vi "Fire WD Event.vi"(8 "error in (no error)":errorcluster, 10 "Completed? (F)":bool, 11 "Search in":refnum<class "Search.lvclass">) -> (0 "error out":errorcluster, 3 "Search out":refnum<class "Search.lvclass">)   [LabVIEW 2016, in "Better Search.lvlib" / "Search.lvclass"]
uses:
  Search.lvclass
  Search Progress.ctl
  Better Search.lvlib
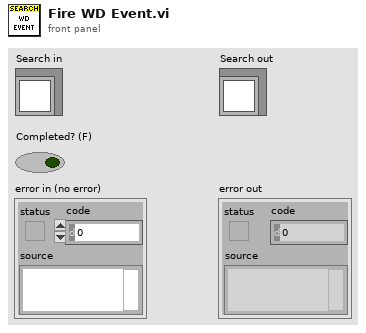
[diagram p1: front panel]
types:
  T1 = typedef "Better Search.lvlib/Search Progress.ctl" = cluster{"Complete":bool, "Label":string}
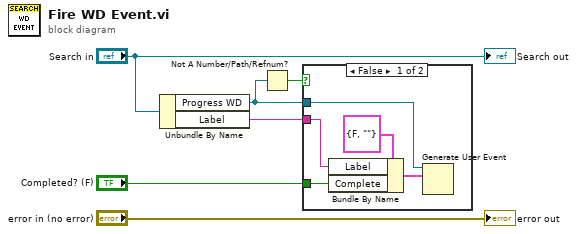
[diagram p0: block diagram]
diagram:
  n1 = Unbundle By Name("Search in") -> ("Progress WD"=w2:refnum<user-event>, "Label"=w4:string)
  n2 = Not A Number/Path/Refnum?(number/path/refnum=w2) -> (NaN/Path/Refnum?=w1:bool)
  n3 = case shown="False" w1 {
    tunnel: w4 -> [w9 _]
    tunnel: "Completed? (F)" -> [w8 _]
    tunnel: w2 -> [w7 _]
    frame False {
      n4 = Bundle By Name(cluster=T1 {"Complete"=FALSE, "Label"=""} ("event data"), "Label"=w9, "Complete"=w8) -> (w10:T1)
      n5 = Generate User Event(user event=w7, event data cluster=w10) -> ()  [unwired: 2 in, 2 out]
    }
    frame True {
    }
  }
  "error out" <- "error in (no error)"
  "Search out" <- "Search in"
